vi "Configure Invert.vi"(8 "error in (no error)":errorcluster, 9 "Invert (T:On)":bool=TRUE, 10 "Channel (1: Channel 1)":u16(ring)=1 items=["Channel 1"=1, "Channel 2"=2, "Channel 3"=3, "Channel 4"=4, "MATH"=5], 11 "VISA resource name":refnum<visa-resource-name>) -> (0 "error out":errorcluster, 3 "VISA resource name out":refnum<visa-resource-name>)   [LabVIEW 2021, in "Siglent SDS 1000 2000 Series.lvlib"]
doc: "Specifies whether you want the oscilloscope turn on the Invert for the specified channel or the MATH function."
uses:
  <instrlib>/Siglent SDS 1000 2000 Series/Siglent SDS 1000 2000 Series.lvlib
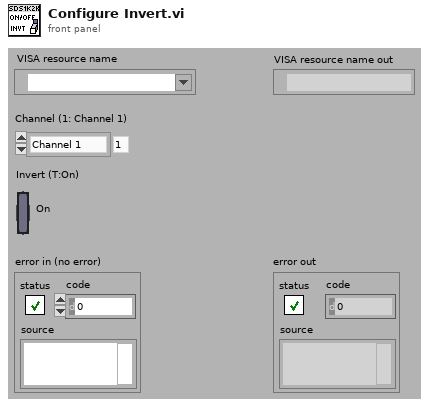
[diagram p1: front panel]
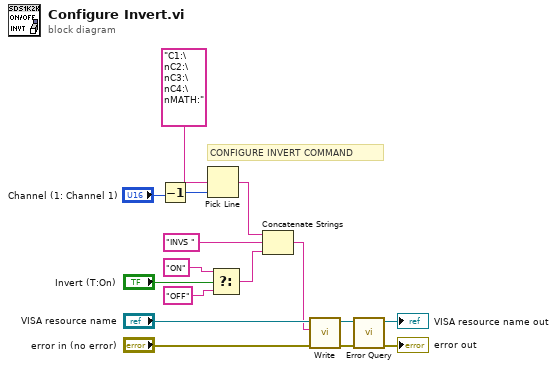
[diagram p0: block diagram]
diagram:
  # "CONFIGURE INVERT COMMAND"
  n1 = Decrement(x="Channel (1: Channel 1)") -> (x-1=w1:u16)
  n2 = Pick Line(multi-line string="C1:\nC2:\nC3:\nC4:\nMATH:", line index=w1) -> (output string=w6:string)  [unwired: 1 in]
  n3 = Select(t="ON", s="Invert (T:On)", f="OFF") -> (s? t:f=w4:string)
  n4 = Concatenate Strings(w6, "INVS ", w4) -> (w3:string)
  n5 = call <instrlib>:"Write.vi"("error in (no error)"="error in (no error)", "Write Buffer"=w3, "VISA resource name"="VISA resource name") -> ("error out"=w11:errorcluster, "VISA resource name out"=w12:refnum<visa-resource-name>)  [unwired: 6 in, 1 out]
  n6 = call <instrlib>:"Error Query.vi"("error in (no error)"=w11, "VISA resource name"=w12) -> ("error out"=→"error out":errorcluster, "VISA resource name out"=→"VISA resource name out":refnum<visa-resource-name>)  [unwired: 6 in, 2 out]
